vi "Read any file waveform --V2.vi"(0 "Input file path":path, 1 "tdms file in":refnum<k34>, 5 "Data window IN":T1={"Start"=39994, "Length"=13169, "Channel numbers"=[0], "Cannel names"=["freq", ""], "Group name"="p"}, 9 "Data File Type":T2(ring), 11 "error in":errorcluster, 12 "(BINARY) 2D number of columns/1D count (all as 1D: -1)":i32=1, 14 "(BINARY) 2D number of rows":i32) -> (3 "tdms file out":refnum<k34>, 4 "Actual input file path":path, 6 "Data out":waveform(dbl)[](array[waveform]), 8 "All Data out":waveform(dbl)[](array[waveform]), 10 "1st channel length":u64, 15 "error out":errorcluster)   [LabVIEW 2021]
uses:
  fft -- data win.ctl
panel:
  out "Header":string
  # "OR"
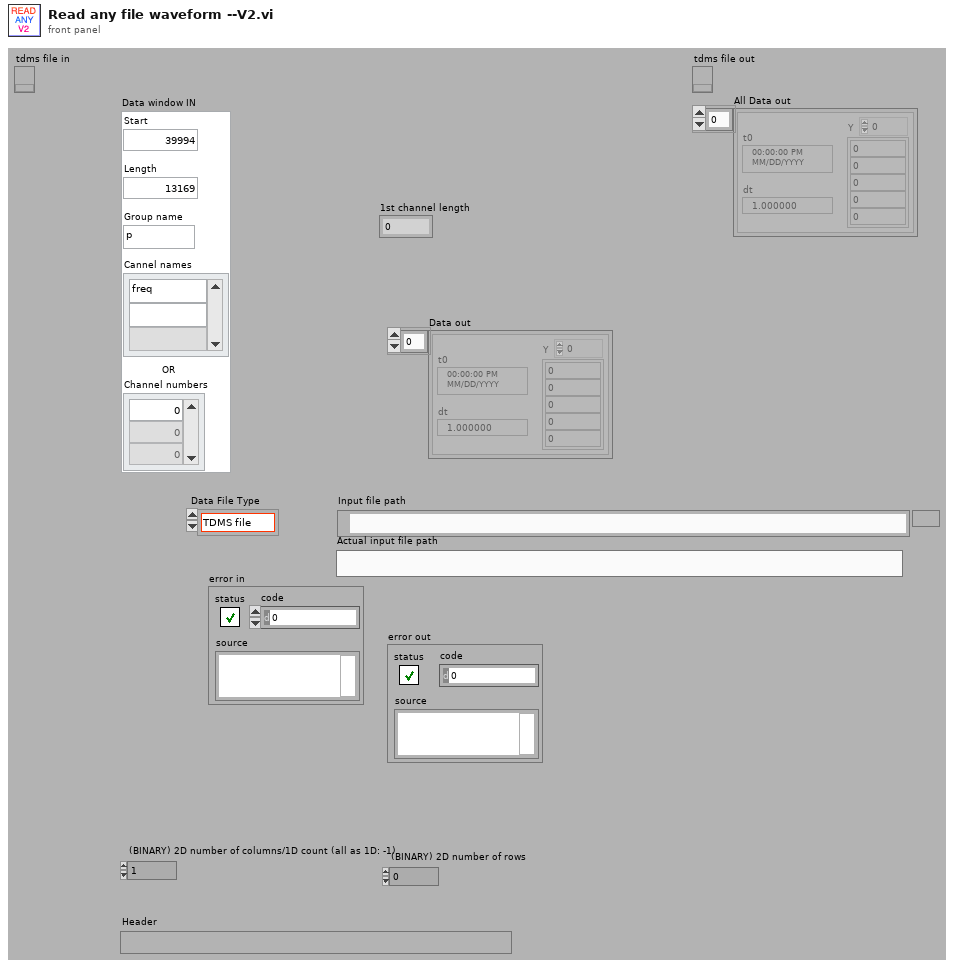
[diagram p1: front panel]
types:
  T1 = typedef "fft -- data win.ctl" = cluster{"Start":i64, "Length":i32, "Channel numbers":i64[], "Cannel names":string[], "Group name":string}
  T2 = enum16{"TDMS file", "Tektronics ISF", "BinF file", "ASCII File", "BinH File", "BinW File", "BINARY File"}
  T3 = enum16{"open", "open or create", "create or replace", "create", "open (read-only)"}
  T4 = cluster{"Version":i16, "Data Representation":enum16{"Undefined", "I8", "I16", "I32", "I64", "U8", "U16", "U32", "U64", "SGL", "DBL", "EXT"}, "# columns (samples per channel)":i64, "# rows (channels)":i64, "# pre-trigger samples":i64, "Sample rate":dbl, "ADC offset":dbl, "Scale factor":dbl}
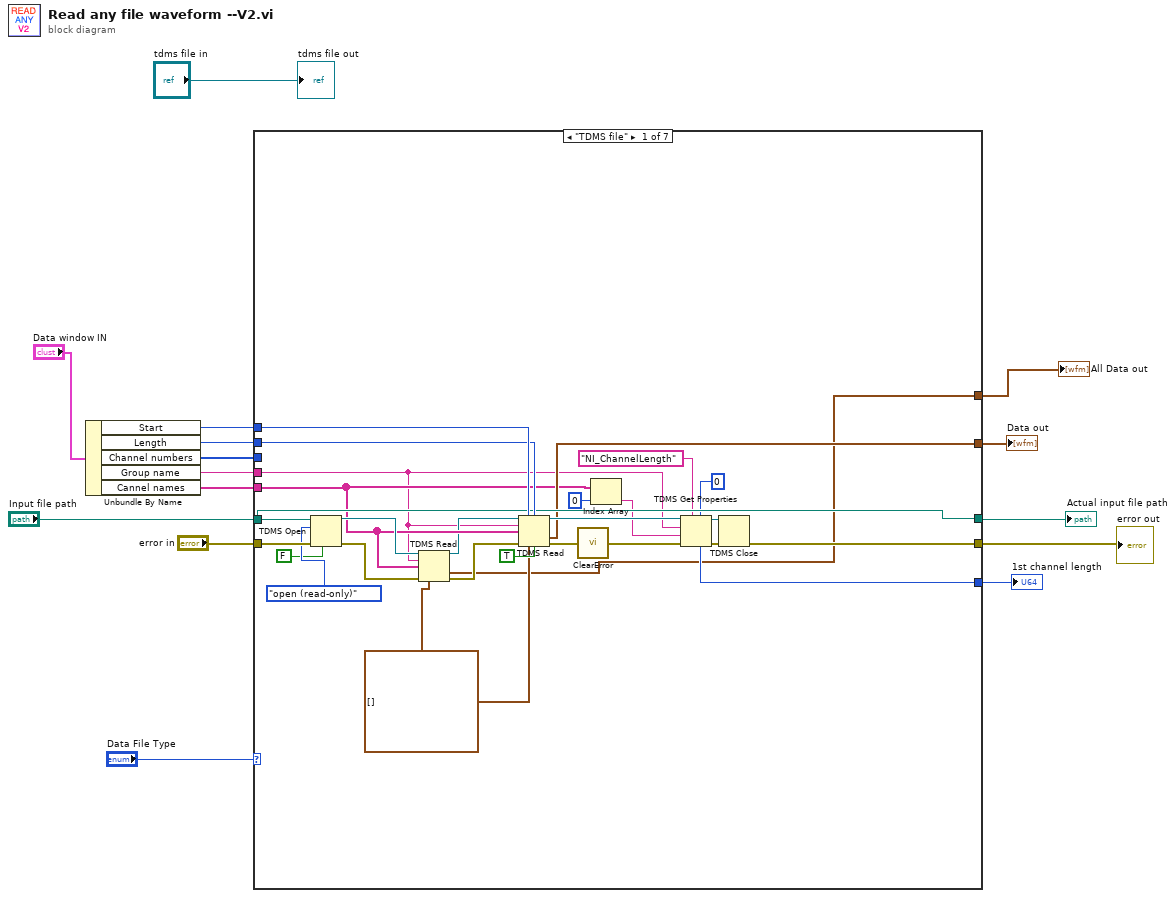
[diagram p0: block diagram]
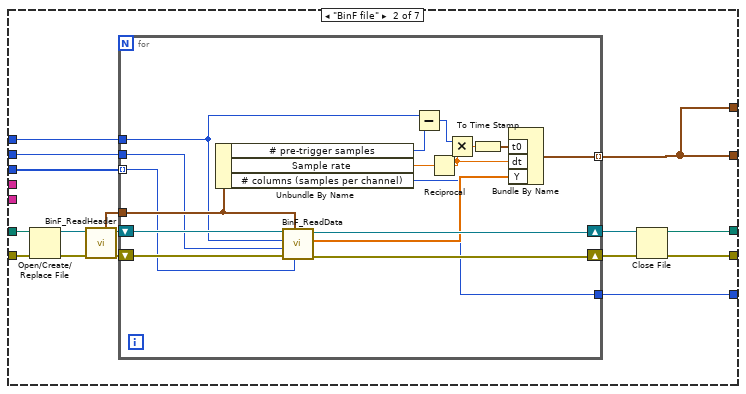
[diagram p2: hidden frame]
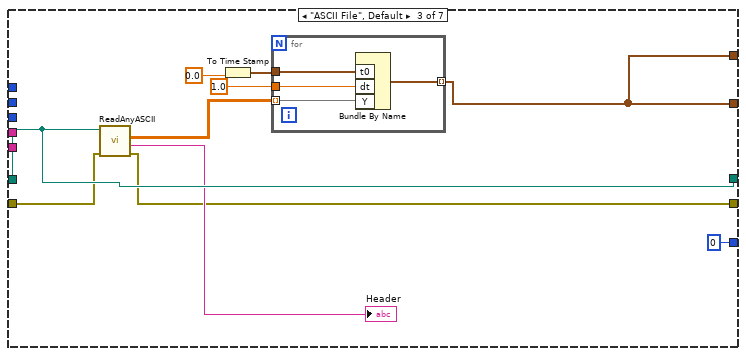
[diagram p3: hidden frame]
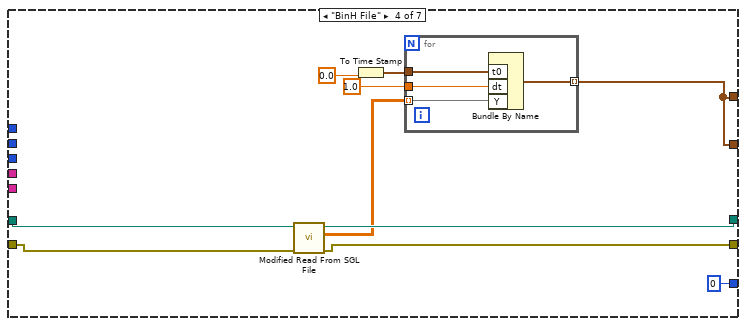
[diagram p4: hidden frame]
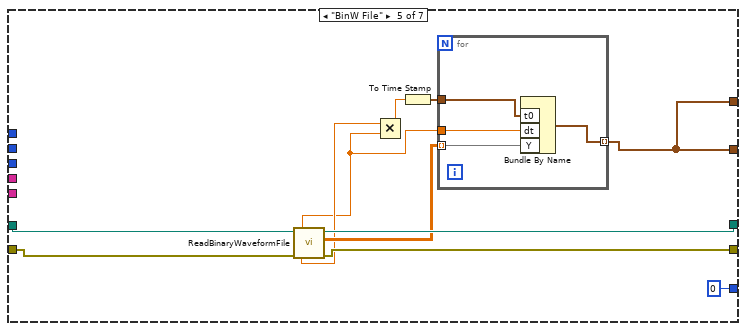
[diagram p5: hidden frame]
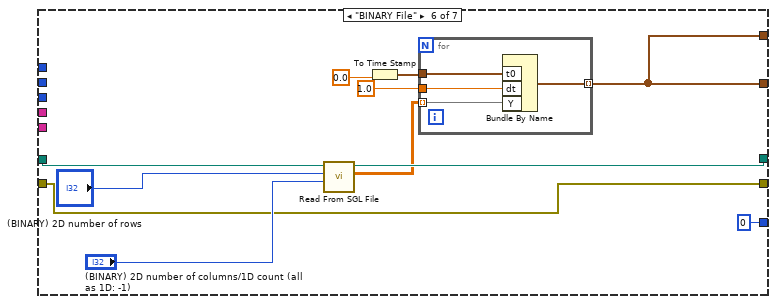
[diagram p6: hidden frame]
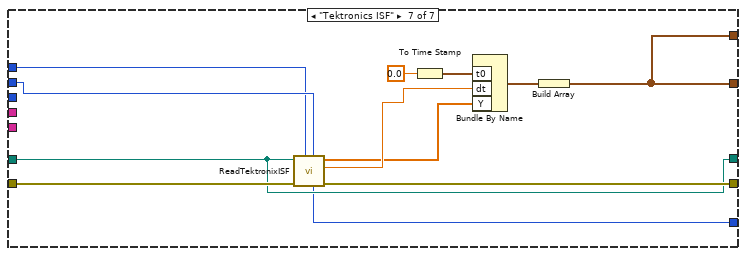
[diagram p7: hidden frame]
diagram:
  n1 = Unbundle By Name("Data window IN") -> ("Start"=w10:i64, "Length"=w9:i32, "Channel numbers"=w11:i64[], "Group name"=w5:string, "Cannel names"=w7:string[])
  n2 = case shown="\"TDMS file\"" "Data File Type" {
    tunnel: "Input file path" -> [w38 w56 w80 w99 w114 w129 w136]
    tunnel: [w38 w48 w80 w98 w113 w128 w136] -> w13
    tunnel: "error in" -> [w42 w55 w78 w97 w112 w122 w139]
    tunnel: [w27 w49 w77 w96 w111 w122 w138] -> w4
    tunnel: w11 -> [_ w47 _ _ _ _ _]
    tunnel: w10 -> [w41 w46 _ _ _ _ w140]
    tunnel: w9 -> [w40 w45 _ _ _ _ w141]
    tunnel: [w29 w43 w76 w90 w104 w119 w134] -> w8
    tunnel: w7 -> [w22 _ _ _ _ _ _]
    tunnel: [w30 w44 u64 0 ("# columns (samples per channel)") u64 0 ("# columns (samples per channel)") u64 0 ("# columns (samples per channel)") u64 0 ("# columns (samples per channel)") w135] -> w6
    tunnel: w5 -> [w16 _ _ _ _ _ _]
    tunnel: [w18 w43 w76 w90 w104 w119 w134] -> w2
    frame "TDMS file" {
      w21 = waveform(dbl)[] []
      n3 = TDMS Open(6:FALSE ("disable buffering (T)"), 8:w42, 10:T3."open (read-only)" ("operation (0:open)"), 11:w38) -> (0:w20:errorcluster, 3:w23:refnum<k34>)  [unwired: 3 in]
      n4 = TDMS Read(0:w23, 5:w16, 7:w22, 11:w20, 12:w21) -> (4:w17:refnum<k34>, 10:w18:waveform(dbl)[], 15:w19:errorcluster)  [unwired: 3 in, 3 out]
      n5 = TDMS Read(0:w17, 1:w41, 2:w40, 5:w16, 7:w22, 11:w19, 12:w21, 13:TRUE ("return channels in file order? (F)")) -> (4:w36:refnum<k34>, 10:w29:waveform(dbl)[], 15:w26:errorcluster)  [unwired: 3 out]
      n6 = call <vilib>:"ClearError.vi"("error in (no error)"=w26) -> ("error out"=w39:errorcluster)
      n7 = Index Array(array=w22, index=0) -> (element=w33:string)
      n8 = TDMS Get Properties(5:u64 0, 7:"NI_ChannelLength" ("property name"), 8:w39, 9:w33, 10:w16, 11:w36) -> (0:w37:errorcluster, 3:w35:refnum<k34>, 4:w30:u64)  [unwired: 3 out]
      n9 = TDMS Close(8:w37, 11:w35) -> (0:w27:errorcluster)  [unwired: 1 out]
    }
    frame "BinF file" {
      n10 = Open/Create/Replace File(file path (use dialog)=w56, error in=w55) -> (refnum out=w57:refnum<file>, error out=w58:errorcluster)  [unwired: 5 out]
      n11 = call "BinF_ReadHeader.vi"("error in"=w58, "refnum"=w57) -> ("error out"=w54:errorcluster, "refnum out"=w53:refnum<file>, "BinF File Settings"=w52:T4)  [unwired: 7 out]
      n12 = for {
        shift-right: [w74] -> w51
        shift-left: w54 -> [w75]
        shift-right: [w72] -> w50
        shift-left: w53 -> [w73]
        tunnel: w52 -> [w65]
        tunnel: w47 -> [w64] mode=indexing
        tunnel: w46 -> [w62]
        tunnel: w45 -> [w63]
        tunnel: [w60] -> w43 mode=indexing
        tunnel: [w59] -> w44
        n13 = Unbundle By Name(w65) -> ("# pre-trigger samples"=w69:i64, "Sample rate"=w67:dbl, "# columns (samples per channel)"=w59:i64)
        n14 = call "BinF_ReadData.vi"("Channel number"=w64, "BinF File Settings"=w65, "error in"=w75, "Length"=w63, "Start"=w62, "refnum"=w73) -> ("error out"=w74:errorcluster, "Channel Data"=w61:sgl[], "refnum out"=w72:refnum<file>)  [unwired: 3 out]
        n15 = Subtract(x=w62, y=w69) -> (x-y=w70:i64)
        n16 = Reciprocal(x=w67) -> (1/x=w68:dbl)
        n17 = Multiply(x=w70, y=w68) -> (x*y=w71:dbl)
        n18 = To Time Stamp(1:w71) -> (0:w66:timestamp)
        n19 = Bundle By Name("t0"=w66, "dt"=w68, "Y"=w61) -> (w60:waveform(sgl))  [unwired: 1 out]
      }
      n20 = Close File(refnum=w50, error in=w51) -> (path=w48:path, error out=w49:errorcluster)
    }
    frame "ASCII File", Default {
      n21 = call "ReadAnyASCII.vi"("error in (no error)"=w78, "file path (dialog if empty)"=w80) -> ("error out"=w77:errorcluster, "Header text"=→"Header":string, "all rows"=w82:dbl[][])  [unwired: 2 in, 5 out]
      n22 = To Time Stamp(1:0.0) -> (0:w84:timestamp)
      n23 = for {
        tunnel: w82 -> [w89] mode=indexing
        tunnel: [w88] -> w76 mode=indexing
        tunnel: w84 -> [w87]
        tunnel: 1.0 -> [w86]
        n24 = Bundle By Name("t0"=w87, "dt"=w86, "Y"=w89) -> (w88:waveform(dbl))  [unwired: 1 out]
      }
    }
    frame "BinH File" {
      n25 = call "Modified Read From SGL File.vi"("error in (no error)"=w97, "file path (dialog if empty)"=w99) -> ("error out"=w96:errorcluster, "2D array"=w92:sgl[][], "new file path (Not A Path if cancelled)"=w98:path)  [unwired: 1 in, 6 out]
      n26 = To Time Stamp(1:0.0) -> (0:w94:timestamp)
      n27 = for {
        tunnel: w92 -> [w103] mode=indexing
        tunnel: [w102] -> w90 mode=indexing
        tunnel: w94 -> [w101]
        tunnel: 1.0 -> [w100]
        n28 = Bundle By Name("t0"=w101, "dt"=w100, "Y"=w103) -> (w102:waveform(sgl))  [unwired: 1 out]
      }
    }
    frame "BinW File" {
      n29 = call "ReadBinaryWaveformFile.vi"("error in (no error)"=w112, "file path (dialog if empty)"=w114) -> ("error out"=w111:errorcluster, "2D array"=w110:sgl[][], "new file path (Not A Path if cancelled)"=w113:path, "Time base"=w109:dbl, "Delay, points"=w106:dbl)  [unwired: 1 in, 4 out]
      n30 = Multiply(x=w109, y=w106) -> (x*y=w108:dbl)
      n31 = To Time Stamp(1:w108) -> (0:w107:timestamp)
      n32 = for {
        tunnel: w110 -> [w117] mode=indexing
        tunnel: [w118] -> w104 mode=indexing
        tunnel: w107 -> [w116]
        tunnel: w106 -> [w115]
        n33 = Bundle By Name("t0"=w116, "dt"=w115, "Y"=w117) -> (w118:waveform(sgl))  [unwired: 1 out]
      }
    }
    frame "BINARY File" {
      n34 = call <vilib>:"Read From SGL File.vi"("2D number of columns/1D count (all as 1D: -1)"="(BINARY) 2D number of columns/1D count (all as 1D: -1)", "2D number of rows"="(BINARY) 2D number of rows", "file path (dialog if empty)"=w129) -> ("2D array"=w126:sgl[][], "new file path (Not A Path if cancelled)"=w128:path)  [unwired: 7 out]
      n35 = To Time Stamp(1:0.0) -> (0:w124:timestamp)
      n36 = for {
        tunnel: w126 -> [w133] mode=indexing
        tunnel: [w132] -> w119 mode=indexing
        tunnel: w124 -> [w131]
        tunnel: 1.0 -> [w130]
        n37 = Bundle By Name("t0"=w131, "dt"=w130, "Y"=w133) -> (w132:waveform(sgl))  [unwired: 1 out]
      }
    }
    frame "Tektronics ISF" {
      n38 = call "ReadTektronixISF.vi"("Length"=w141, "Start"=w140, "error in (no error)"=w139, "Path"=w136) -> ("error out"=w138:errorcluster, "dt"=w145:dbl, "Data"=w137:dbl[], "Total number of points"=w135:u64)  [unwired: 4 out]
      n39 = To Time Stamp(1:0.0) -> (0:w142:timestamp)
      n40 = Bundle By Name("t0"=w142, "dt"=w145, "Y"=w137) -> (w144:waveform(dbl))  [unwired: 1 out]
      n41 = Build Array(w144) -> (w134:waveform(dbl)[])
    }
  }
  "Actual input file path" <- w13
  "error out" <- w4
  "Data out" <- w8
  "1st channel length" <- w6
  "All Data out" <- w2
  "tdms file out" <- "tdms file in"
